vi "destroyTempControllerFrontEndEvents.vi"(8 "error in (no error)":errorcluster, 10 "tempControllerFrontEndEvents":T1, 11 "CameraEventsManger in":refnum<class "CameraEventsManger.lvclass">) -> (0 "error out":errorcluster, 3 "CameraEventsManger out":refnum<class "CameraEventsManger.lvclass">)   [LabVIEW 2011, in "Tools.lvlib" / "Settings.lvlib" / "CameraEventsManger.lvclass"]
uses:
  CameraEventsManger.lvclass
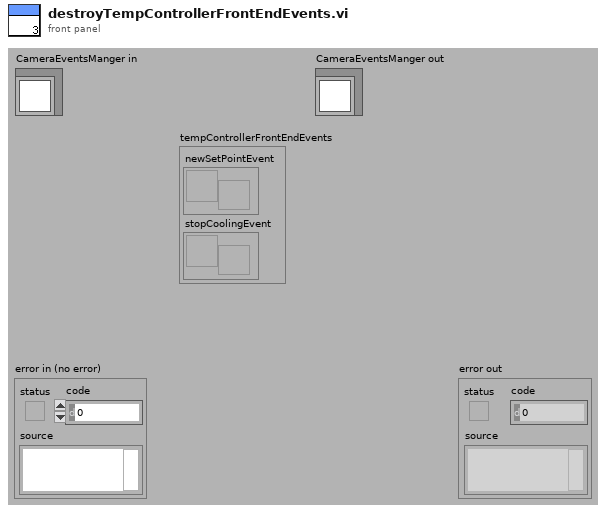
[diagram p1: front panel]
types:
  T1 = cluster{"newSetPointEvent":refnum<user-event>, "stopCoolingEvent":refnum<user-event>}
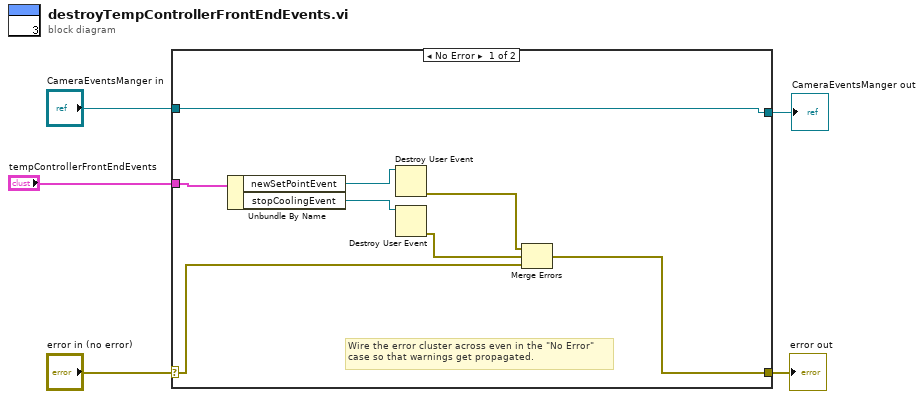
[diagram p0: block diagram]
diagram:
  n1 = case shown="No Error" "error in (no error)" {
    selector: "error in (no error)" -> [w8 w15]
    tunnel: [w7 w15] -> w4
    tunnel: "CameraEventsManger in" -> [w6 w14]
    tunnel: "tempControllerFrontEndEvents" -> [w13 _]
    tunnel: [w6 w14] -> w1
    frame No Error {
      # "Wire the error cluster across even in the \"No Error\"\ncase so that warnings get propagated."
      n2 = Unbundle By Name(w13) -> ("newSetPointEvent"=w12:refnum<user-event>, "stopCoolingEvent"=w11:refnum<user-event>)
      n3 = Destroy User Event(user event=w12) -> (error out=w10:errorcluster)  [unwired: 1 in]
      n4 = Destroy User Event(user event=w11) -> (error out=w9:errorcluster)  [unwired: 1 in]
      n5 = Merge Errors(w10, w9, w8) -> (w7:errorcluster)
    }
    frame Error {
    }
  }
  "error out" <- w4
  "CameraEventsManger out" <- w1
